vi "init.vi"(8 "error in (no error)":errorcluster, 11 "EnccoderConverter in":refnum<class "EncoderConverterTC.lvclass">) -> (0 "error out":errorcluster, 3 "EnccoderConverter out":refnum<class "EncoderConverterTC.lvclass">)   [LabVIEW 2013, in "EncoderConverterTC.lvclass"]
uses:
  EncoderConverterTC.lvclass
  <userlib>/Common/Devices/EncoderConverter/Config/EncoderConverter.ctl
  <userlib>/Common/Devices/EncoderConverter/EncoderConverter/EncoderConverter.lvclass/EncoderConverter.ctl
  <userlib>/Common/Devices/EncoderConverter/EncoderConverter/EncoderConverter.lvclass
  ConfigurationThisComponent/ConfigurationThisComponent.lvclass
  <userlib>/Common/Devices/EncoderConverter/EncoderConverter.lvlib
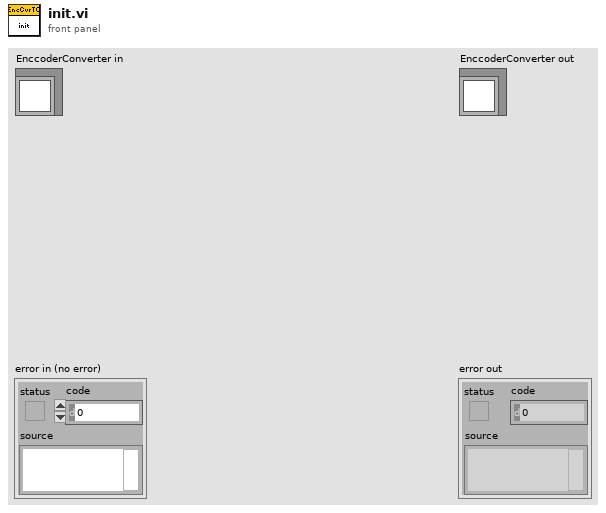
[diagram p1: front panel]
types:
  T1 = typedef "EncoderConverter.lvlib/EncoderConverter.ctl" = cluster{"Distance Per Count":dbl[unit]}
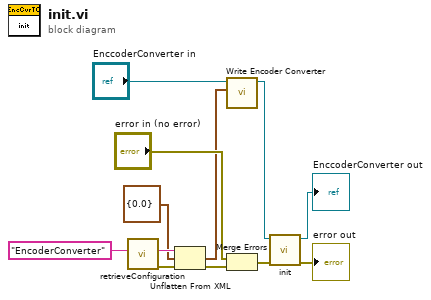
[diagram p0: block diagram]
diagram:
  n1 = call "retrieveConfiguration.vi"("configName"="EncoderConverter") -> ("error out"=w8:errorcluster, "xmlConfig"=w9:string)  [unwired: 8 in, 1 out]
  n2 = Unflatten From XML(xml string=w9, type=T1 {"Distance Per Count"=0.0} ("Encoder"), error in (no error)=w8) -> (value=w3:T1, error out=w5:errorcluster)
  n3 = call <userlib>:"Write Encoder Converter.vi"("Enccoder Converter"=w3, "EncoderConverter in"="EnccoderConverter in") -> ("EncoderConverter out"=w1:refnum<class "EncoderConverterTC.lvclass">)  [unwired: 9 in]
  n4 = Merge Errors("error in (no error)", w5) -> (w4:errorcluster)
  n5 = call-parent "init.vi"("error in (no error)"=w4, "EnccoderConverter in"=w1) -> ("error out"=→"error out":errorcluster, "EnccoderConverter out"=→"EnccoderConverter out":refnum<class "EncoderConverterTC.lvclass">)  [unwired: 8 in]
